vi "Process.vi"(11 "Config":T1) -> ()   [LabVIEW 2020, in "RTAF.lvlib" / "Alarms Handler Actor.lvclass"]
uses:
  Alarms Handler Actor.lvclass
  Config.ctl
  Base Actor/Actor/Actor.lvclass/Actor.ctl
  Base Actor/Sequencer/Sequencer.lvclass/Sequencer.ctl
  Alarms Handler Actor.lvclass/Alarms Handler Actor.ctl
  <vilib>/Utility/High Resolution Relative Seconds.vi
  C:/dev/PGS/2001 - TBCM/Source/RT/RTAF/Source/RTAF/Actors/Base Actor/Actor/Actor.lvclass
  Base Actor/Actor/Actor.lvclass
  Logger/API/Logger Actor API.lvclass
  RTAF.lvlib
panel:
  in  "Acknowledge":bool
  out "Number Of Alarms":i32
  out "Alarms":errorcluster[](array[cluster])
  out "Iteration":i32
  in  "Tick Period [ms]":i32=5 min=2 step=1
  out "Tick Period [s]":dbl format="%.1p"
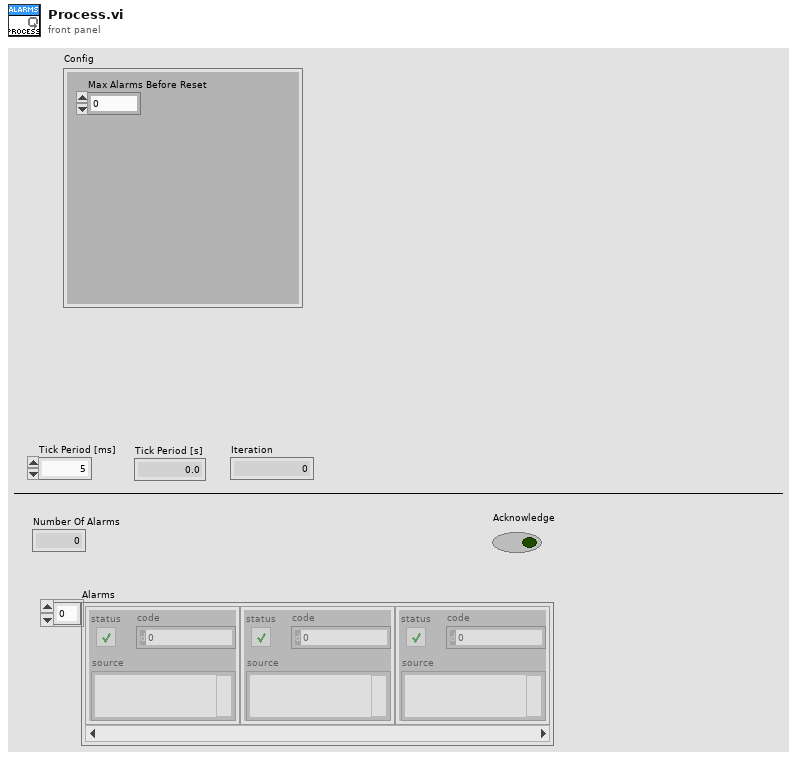
[diagram p1: front panel]
types:
  T1 = typedef "RTAF.lvlib/Alarms Handler Actor.lvclass/Config.ctl" = cluster{"Max Alarms Before Reset":i32}
  T2 = enum32{"Invalid", "Standard", "Closed", "Hidden", "Minimized", "Maximized"}
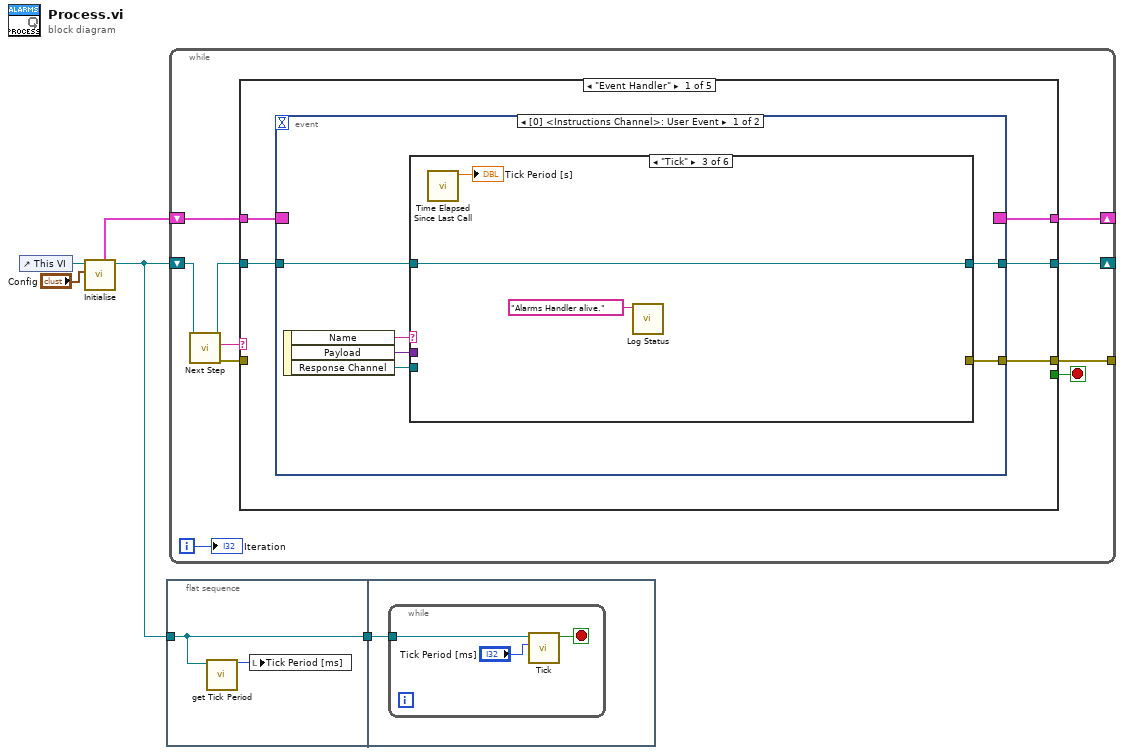
[diagram p0: block diagram]
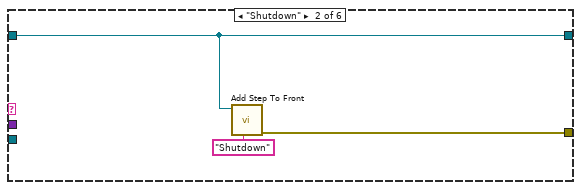
[diagram p3: hidden frame]
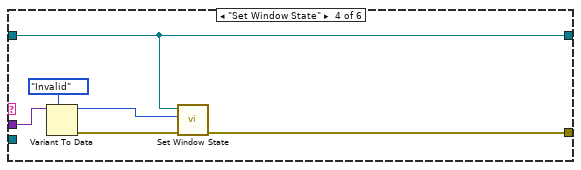
[diagram p4: hidden frame]
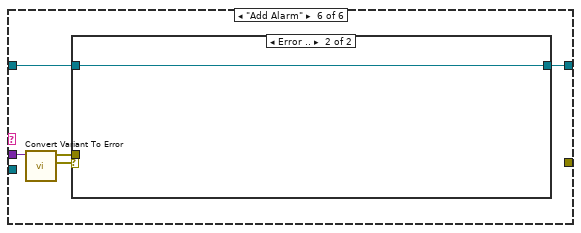
[diagram p6: hidden frame]
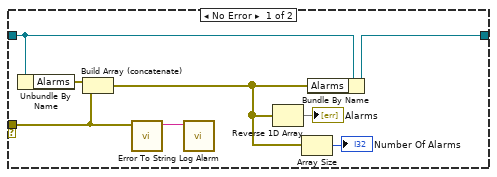
[diagram p7: hidden frame]
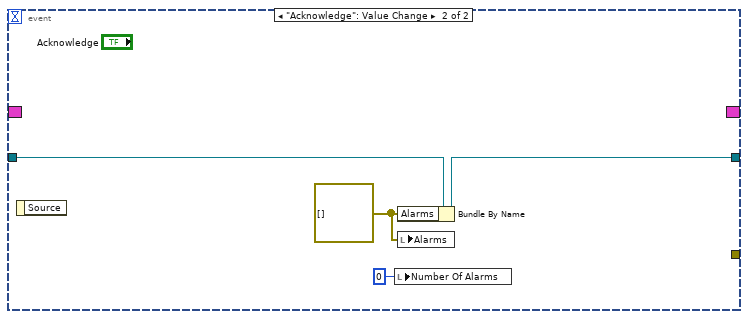
[diagram p8: hidden frame]
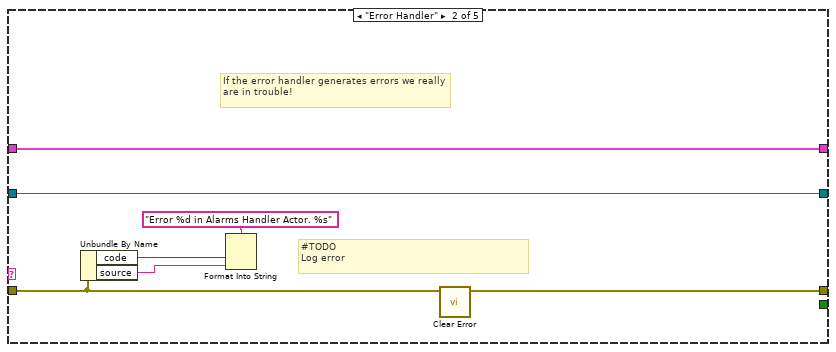
[diagram p9: hidden frame]
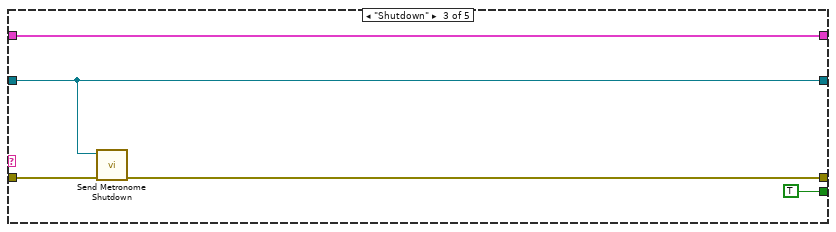
[diagram p10: hidden frame]
diagram:
  n1 = control-ref of="This VI"() -> (w2:refnum<vi>)
  n2 = call "Initialise.vi"("Config"="Config", "Process"=w2) -> ("Actor out"=w4:refnum<class "Alarms Handler Actor.lvclass">, "Mailboxes"=w3:cluster{"Mailbox":refnum<event-registration>})  [unwired: 7 in, 1 out]
  n3 = flat-sequence {
    tunnel: w4 -> [w7]
    tunnel: [w7] -> w5
    tunnel: w5 -> [w8]
    frame #0 {
      n4 = call "get Tick Period.vi"("Actor in"=w7) -> ("Tick Period [ms]"=w6:i32)  [unwired: 10 in]
      n5 = local write "Tick Period [ms]"(w6) -> ()
    }
    frame #1 {
      n6 = while {
        tunnel: w8 -> [w11]
        stop <- w9 stop-if-true
        n7 = call "Tick.vi"("Tick Period [ms]"="Tick Period [ms]", "Actor in"=w11) -> ("Shutdown"=w9:bool)  [unwired: 9 in]
      }
    }
  }
  n8 = while {
    shift-right: [w20] -> _
    shift-left: w4 -> [w17]
    tunnel: [w19] -> _
    shift-right: [w12] -> _
    shift-left: w3 -> [w21]
    i -> [w13]
    stop <- w14 stop-if-true
    n9 = call "Next Step.vi"("Actor in"=w17) -> ("error out"=w18:errorcluster, "Next Step"=w15:string, "Actor out"=w16:refnum<class "Alarms Handler Actor.lvclass">)  [unwired: 8 in]
    n10 = case shown="\"Event Handler\"" w15 {
      tunnel: w21 -> [w26 w70 w72 w77 w80]
      tunnel: [_ _ TRUE _ _] -> w14
      tunnel: w16 -> [w25 w71 w75 w79 w82]
      tunnel: [w24 w71 w75 w79 w82] -> w20
      tunnel: [w23 w65 w74 w78 w81] -> w19
      tunnel: w18 -> [_ w66 w73 w78 w81]
      tunnel: [w22 w70 w72 w77 w80] -> w12
      frame "Event Handler" {
        n11 = event shown="[0] <Instructions Channel>: User Event" {
          selector: w26 -> [_ _]
          dyn-events: [_ _] -> w22
          timeout: _ -> [_ _]
          tunnel: w25 -> [w30 w63]
          tunnel: [w29 w64] -> w24
          tunnel: [w27 _] -> w23
          event User Event {
            n12 = event-data() -> ("Name"=w32:string, "Payload"=w31:variant, "Response Channel"=w28:refnum<notifier>)  [unwired: 1 in]
            n13 = case shown="\"Tick\"" w32 {
              tunnel: w31 -> [_ _ _ w45 _ w49]
              tunnel: w30 -> [w33 w36 w39 w42 w46 w50]
              tunnel: [w33 w36 w39 w42 w46 w51] -> w29
              tunnel: w28 -> [_ _ _ _ _ _]
              tunnel: [_ w35 _ w43 _ _] -> w27
              frame Default {
              }
              frame "Shutdown" {
                n14 = call "Add Step To Front.vi"("Step Name"="Shutdown", "Actor in"=w36) -> ("error out"=w35:errorcluster)  [unwired: 9 in]
              }
              frame "Tick" {
                n15 = call "Time Elapsed Since Last Call.vi"() -> ("Time Elapsed Since Last Call [s]"=→"Tick Period [s]":dbl)  [unwired: 11 in]
                n16 = call "Log Status.vi"("Message"="Alarms Handler alive.") -> ()  [unwired: 10 in, 1 out]
              }
              frame "Set Window State" {
                n17 = Variant To Data(type=T2."Invalid", Variant=w45) -> (data=w41:T2, error out=w44:errorcluster)  [unwired: 1 in]
                n18 = call "Set Window State.vi"("error in (no error)"=w44, "State"=w41, "Actor in"=w42) -> ("error out"=w43:errorcluster)  [unwired: 8 in]
              }
              frame "----------------------------------" {
              }
              frame "Add Alarm" {
                n19 = call "Convert Variant To Error.vi"("Variant"=w49) -> ("error out"=w47:errorcluster, "Error"=w48:errorcluster)  [unwired: 9 in]
                n20 = case shown="Error .." w47 {
                  tunnel: [w59 w60] -> w51
                  tunnel: w50 -> [w58 w60]
                  tunnel: w48 -> [w53 _]
                  frame No Error {
                    n21 = Unbundle By Name(w58) -> ("Alarms"=w57:errorcluster[])
                    n22 = Build Array (concatenate)(w57, w53) -> (w55:errorcluster[])
                    n23 = call "Error To String.vi"("error in (no error)"=w53) -> ("String"=w52:string)  [unwired: 10 in]
                    n24 = call "Log Alarm.vi"("Message"=w52) -> ()  [unwired: 10 in, 1 out]
                    n25 = Reverse 1D Array(array=w55) -> (reversed array=→"Alarms":errorcluster[])
                    n26 = Array Size(array=w55) -> (size(s)=→"Number Of Alarms":i32)
                    n27 = Bundle By Name(cluster=w58, "Alarms"=w55) -> (w59:refnum<class "Alarms Handler Actor.lvclass">)
                  }
                  frame Error {
                  }
                }
              }
            }
          }
          event "Acknowledge": Value Change {
            w62 = errorcluster[] [] ("Alarms")
            n28 = event-data() -> ()  [unwired: 1 in, 1 out]
            n29 = local write "Number Of Alarms"(0 ("Number Of Alarms")) -> ()
            n30 = Bundle By Name(cluster=w63, "Alarms"=w62) -> (w64:refnum<class "Alarms Handler Actor.lvclass">)
            n31 = local write "Alarms"(w62) -> ()
          }
        }
      }
      frame "Error Handler" {
        # "#TODO\nLog error"
        # "If the error handler generates errors we really are in trouble!"
        n32 = Unbundle By Name(w66) -> ("code"=w68:i32, "source"=w67:string)
        n33 = Format Into String(format string="Error %d in Alarms Handler Actor. %s", w68, w67) -> ()  [unwired: 2 in, 2 out]
        n34 = call "Clear Error.vi"("error in (no error)"=w66) -> ("error out"=w65:errorcluster)  [unwired: 6 in]
      }
      frame "Shutdown" {
        n35 = call "Send Metronome Shutdown.vi"("error in (no error)"=w73, "Actor in"=w75) -> ("error out"=w74:errorcluster)  [unwired: 9 in]
      }
      frame "Unhandled Step", Default {
      }
      frame "-----------------------------------" {
      }
    }
    "Iteration" <- w13
  }
